vi "FFT_Tester.vi"   [LabVIEW 2015]
uses:
  <vilib>/rvi/Analysis/measure/FFT/XNode/niFpgaFFT.xnode
  <vilib>/rvi/Analysis/measure/FFT/XNode/niFpgaFFTButterflyDelays.ctl
  <vilib>/fxp/LVFixedPointQuantizationPolicyTypeDef.ctl
  <vilib>/rvi/Analysis/measure/FFT/simModelSupport/niFpgaFFTSimDfxp.ctl
  <vilib>/rvi/Analysis/measure/FFT/simModelSupport/niFpgaFFTSimArithmeticProperties.ctl
  <vilib>/rvi/Analysis/measure/FFT/simModelSupport/niFPGA FFT Sim Types.ctl
  <vilib>/rvi/Analysis/measure/FFT/simModelSupport/niFPGA FFT Sim Stream Group Properties.ctl
  <vilib>/rvi/Analysis/measure/FFT/simModelSupport/niFPGA FFT Streaming Sim Properties.ctl
  <vilib>/rvi/Analysis/measure/FFT/simModelSupport/niFpgaFFTSimModelStreamingCore.vi
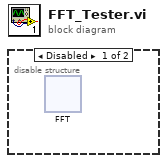
[diagram p0: block diagram]
diagram:
  n1 = disable-structure shown="Disabled" {
    frame Disabled {
      n2 = xnode "FFT"() -> ()  [unwired: 5 in, 5 out]
    }
    frame Enabled {
    }
  }
